vi "Get ACK.vi"(8 "error in (no error)":errorcluster, 11 "niDTS Comm String in":refnum<class "niDTS Comm String.lvclass">) -> (0 "error out":errorcluster, 2 "ACK":string, 3 "niDTS Comm String out":refnum<class "niDTS Comm String.lvclass">)   [LabVIEW 2015, in "niDTS CommLib.lvlib" / "niDTS Comm String.lvclass"]
uses:
  niDTS Comm String.lvclass
  niDTS Comm String.lvclass/niDTS Comm String.ctl
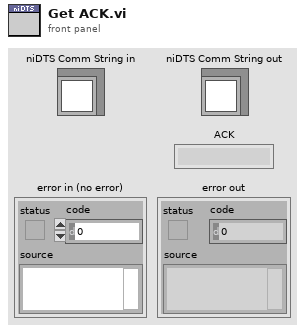
[diagram p1: front panel]
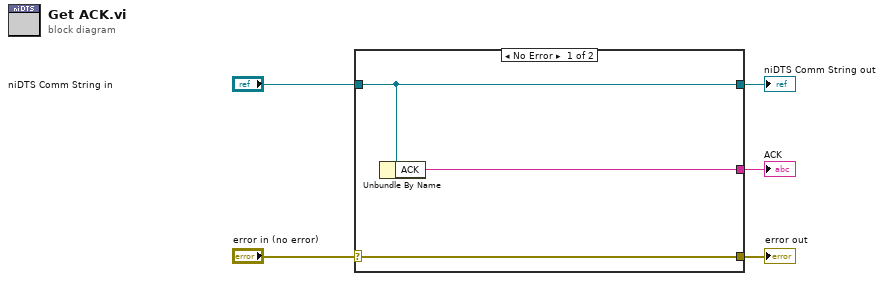
[diagram p0: block diagram]
diagram:
  n1 = case shown="No Error" "error in (no error)" {
    selector: "error in (no error)" -> [w8 w9]
    tunnel: [w8 w9] -> w4
    tunnel: [w7 w10] -> w2
    tunnel: "niDTS Comm String in" -> [w7 w10]
    tunnel: [w6 _] -> w1
    frame No Error {
      n2 = Unbundle By Name(w7) -> ("ACK"=w6:string)
    }
    frame Error {
    }
  }
  "error out" <- w4
  "niDTS Comm String out" <- w2
  "ACK" <- w1
